vi "Element Editor Panels.vi"() -> (2 "Panels":T1(c390))   [LabVIEW 2020, in "VolatusGUIEditor.lvlib"]
uses:
  VolatusGUIEditor.lvlib
  VolatusGUIEditorCore/ElementEditorPanel/ElementEditorPanel.lvclass
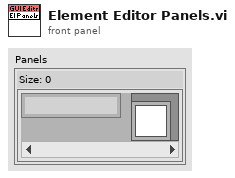
[diagram p1: front panel]
types:
  T1 = map{string, refnum<class "ElementEditorPanel.lvclass">}
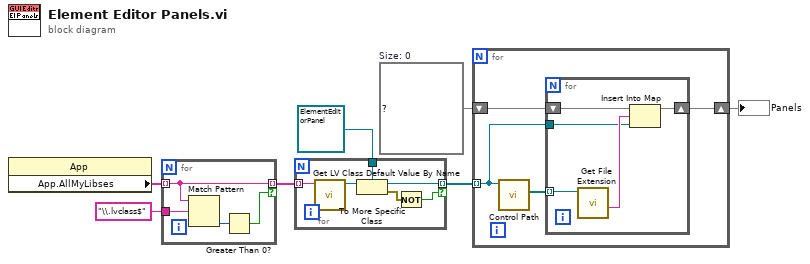
[diagram p0: block diagram]
diagram:
  w2 = T1 {}  # Size: 0
  n1 = property class="App"() -> ("App.AllMyLibses"=w7:string[])  [unwired: 2 in, 2 out]
  n2 = for {
    tunnel: w7 -> [w10] mode=indexing
    tunnel: "\\.lvclass$" -> [w11]
    tunnel: [w10] -> w5 mode=indexing if=w8
    n3 = Match Pattern(string=w10, regular expression=w11) -> (offset past match=w9:i32)  [unwired: 1 in, 3 out]
    n4 = Greater Than 0?(x=w9) -> (x > 0?=w8:bool)
  }
  n5 = for {
    tunnel: w5 -> [w17] mode=indexing
    tunnel: refnum<class "ElementEditorPanel.lvclass"> refnum ("VolatusGUIControls.lvlib:ElementEditorPanel.lvclass") -> [w15]
    tunnel: [w14] -> w3 mode=indexing if=w12
    n6 = call <vilib>:"Get LV Class Default Value By Name.vi"("class name"=w17) -> ("object"=w16:refnum<class>)  [unwired: 9 in, 1 out]
    n7 = To More Specific Class(target class=w15, reference=w16) -> (specific class reference=w14:refnum<class "ElementEditorPanel.lvclass">, error out=w13:errorcluster)  [unwired: 1 in]
    n8 = Not(x=w13) -> (.not. x?=w12:bool)
  }
  n9 = for {
    tunnel: w3 -> [w19] mode=indexing
    shift-right: [w18] -> w1
    shift-left: w2 -> [w20]
    n10 = call-dynamic "Control Path.vi"("ElementEditorPanel in"=w19) -> ("Control Paths"=w21:path[])  [unwired: 10 in]
    n11 = for {
      tunnel: w21 -> [w26] mode=indexing
      tunnel: w19 -> [w23]
      shift-right: [w22] -> w18
      shift-left: w20 -> [w25]
      n12 = call <vilib>:"Get File Extension.vi"("file"=w26) -> ("filename without extension"=w24:string)  [unwired: 6 in, 4 out]
      n13 = Insert Into Map(map in=w25, key=w24, value=w23) -> (map out=w22:T1)  [unwired: 2 out]
    }
  }
  "Panels" <- w1
